vi "isDisabled.vi"(8 "error in (no error)":errorcluster, 11 "Category in":refnum<class "Category.lvclass">) -> (0 "error out":errorcluster, 2 "Disabled?":bool, 3 "Category out":refnum<class "Category.lvclass">)   [LabVIEW 2020, in "Category.lvclass"]
uses:
  Category.lvclass
  Category.lvclass/Category.ctl
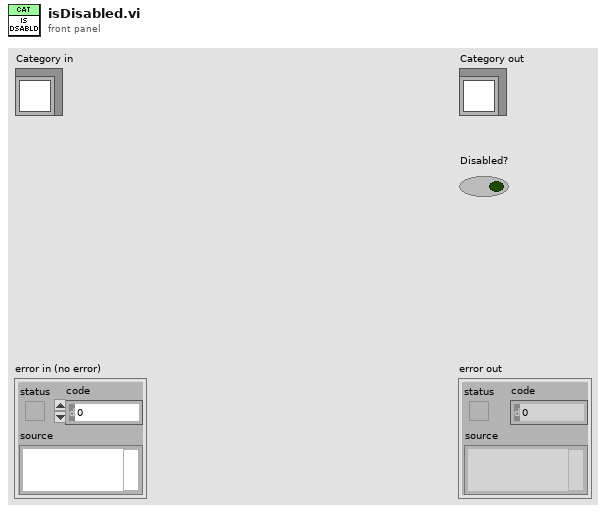
[diagram p1: front panel]
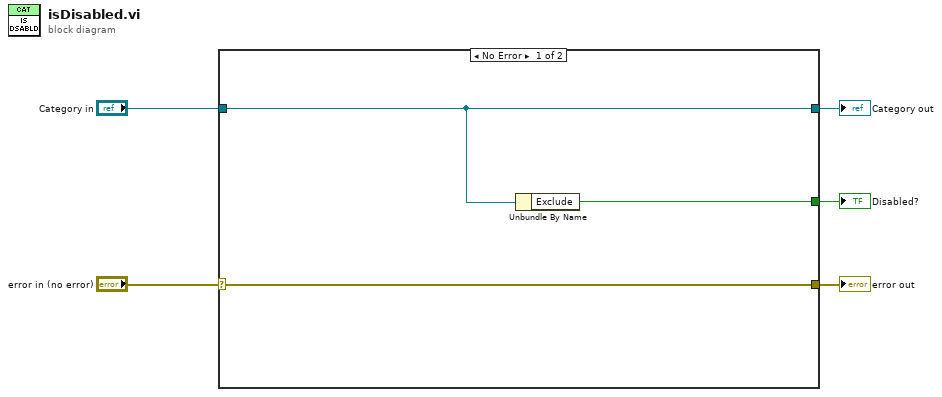
[diagram p0: block diagram]
diagram:
  n1 = case shown="No Error" "error in (no error)" {
    selector: "error in (no error)" -> [w8 w10]
    tunnel: [w8 w10] -> w4
    tunnel: [w7 w9] -> w2
    tunnel: "Category in" -> [w7 w9]
    tunnel: [w6 _] -> w1
    frame No Error {
      n2 = Unbundle By Name(w7) -> ("Exclude"=w6:bool)
    }
    frame Error {
    }
  }
  "error out" <- w4
  "Category out" <- w2
  "Disabled?" <- w1
